vi "JoyStick.vi"(11 "Enum":enum16{"Init", "Run", "End"}(ring)) -> (0 "JoyStick 4":T2, 1 "JoyStick 3":T2, 2 "JoyStick 2":T2, 3 "JoyStick 1":T2)   [LabVIEW 2011]
uses:
  <vilib>/Rock Robotics/WPI/Joystick/WPI_JoystickButtonState.ctl
  <vilib>/Rock Robotics/WPI/Joystick/WPI_JoystickDeviceEnum.ctl
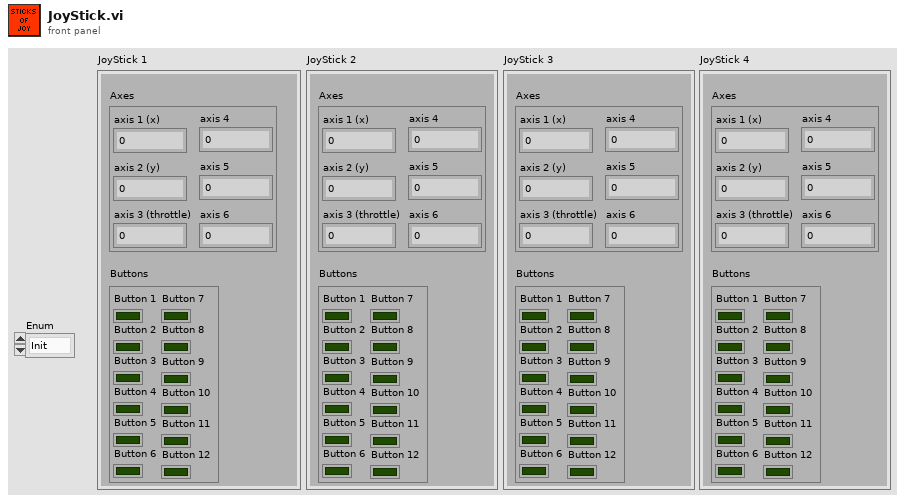
[diagram p1: front panel]
types:
  T1 = typedef "WPI_JoystickButtonState.ctl" = cluster{"Button 1":bool, "Button 2":bool, "Button 3":bool, "Button 4":bool, "Button 5":bool, "Button 6":bool, "Button 7":bool, "Button 8":bool, "Button 9":bool, "Button 10":bool, "Button 11":bool, "Button 12":bool}
  T2 = cluster{"Buttons":T1, "Axes":cluster{"axis 1 (x)":dbl, "axis 2 (y)":dbl, "axis 3 (throttle)":dbl, "axis 4":dbl, "axis 5":dbl, "axis 6":dbl}}
  T3 = typedef "WPI_JoystickDeviceEnum.ctl" = enum16{"USB 1", "USB 2", "USB 3", "USB 4", "Kinect 1", "Kinect 2"}
  T4 = typedef "WPI_JoystickDevRef.ctl" = cluster{"Device":T3}
  T5 = cluster{"axis 1 (x)":dbl, "axis 2 (y)":dbl, "axis 3 (throttle)":dbl, "axis 4":dbl, "axis 5":dbl, "axis 6":dbl}
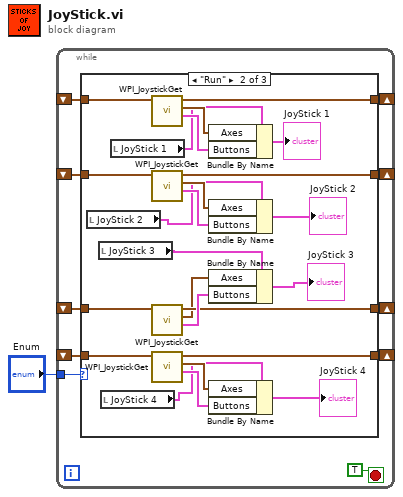
[diagram p0: block diagram]
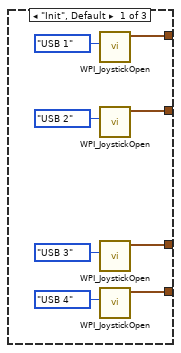
[diagram p2: hidden frame]
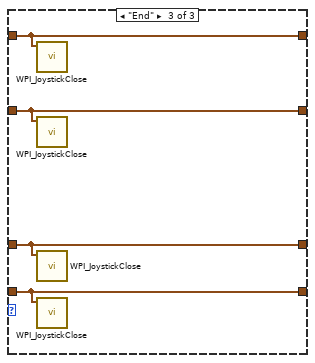
[diagram p3: hidden frame]
diagram:
  n1 = while {
    tunnel: "Enum" -> [w11]
    shift-right: [w10] -> _
    shift-left: _ -> [w8]
    shift-right: [w9] -> _
    shift-left: _ -> [w7]
    shift-right: [w5] -> _
    shift-left: _ -> [w4]
    shift-right: [w6] -> _
    shift-left: _ -> [w3]
    stop <- TRUE stop-if-true
    n2 = case shown="\"Run\"" w11 {
      tunnel: [w19 w42 w47] -> w10
      tunnel: [w18 w30 w46] -> w9
      tunnel: w8 -> [_ w43 w47]
      tunnel: w7 -> [_ w29 w46]
      tunnel: [w17 w26 w44] -> w6
      tunnel: [w16 w33 w45] -> w5
      tunnel: w4 -> [_ w34 w45]
      tunnel: w3 -> [_ w28 w44]
      frame "Init", Default {
        n3 = call <vilib>:"WPI_JoystickOpen.vi"("JoystickDevice"=WPI_JoystickDeviceEnum."USB 1") -> ("JoystickDevRef"=w19:T4)  [unwired: 10 in]
        n4 = call <vilib>:"WPI_JoystickOpen.vi"("JoystickDevice"=WPI_JoystickDeviceEnum."USB 2") -> ("JoystickDevRef"=w18:T4)  [unwired: 10 in]
        n5 = call <vilib>:"WPI_JoystickOpen.vi"("JoystickDevice"=WPI_JoystickDeviceEnum."USB 3") -> ("JoystickDevRef"=w16:T4)  [unwired: 10 in]
        n6 = call <vilib>:"WPI_JoystickOpen.vi"("JoystickDevice"=WPI_JoystickDeviceEnum."USB 4") -> ("JoystickDevRef"=w17:T4)  [unwired: 10 in]
      }
      frame "Run" {
        n7 = local read "JoyStick 2"() -> (w24:T2)
        n8 = local read "JoyStick 3"() -> (w21:T2)
        n9 = local read "JoyStick 4"() -> (w20:T2)
        n10 = local read "JoyStick 1"() -> (w39:T2)
        n11 = call <vilib>:"WPI_JoystickGet.vi"("JoystickDevRef"=w43) -> ("Buttons"=w40:T1, "Axes"=w41:T5, "JoystickDevRef"=w42:T4)  [unwired: 4 in]
        n12 = call <vilib>:"WPI_JoystickGet.vi"("JoystickDevRef"=w29) -> ("Buttons"=w36:T1, "Axes"=w31:T5, "JoystickDevRef"=w30:T4)  [unwired: 4 in]
        n13 = call <vilib>:"WPI_JoystickGet.vi"("JoystickDevRef"=w34) -> ("Buttons"=w35:T1, "Axes"=w32:T5, "JoystickDevRef"=w33:T4)  [unwired: 4 in]
        n14 = call <vilib>:"WPI_JoystickGet.vi"("JoystickDevRef"=w28) -> ("Buttons"=w37:T1, "Axes"=w27:T5, "JoystickDevRef"=w26:T4)  [unwired: 4 in]
        n15 = Bundle By Name(cluster=w39, "Axes"=w41, "Buttons"=w40) -> (→"JoyStick 1":T2)
        n16 = Bundle By Name(cluster=w24, "Axes"=w31, "Buttons"=w36) -> (→"JoyStick 2":T2)
        n17 = Bundle By Name(cluster=w21, "Axes"=w32, "Buttons"=w35) -> (→"JoyStick 3":T2)
        n18 = Bundle By Name(cluster=w20, "Axes"=w27, "Buttons"=w37) -> (→"JoyStick 4":T2)
      }
      frame "End" {
        n19 = call <vilib>:"WPI_JoystickClose.vi"("JoystickDevRef"=w47) -> ()  [unwired: 11 in]
        n20 = call <vilib>:"WPI_JoystickClose.vi"("JoystickDevRef"=w46) -> ()  [unwired: 11 in]
        n21 = call <vilib>:"WPI_JoystickClose.vi"("JoystickDevRef"=w45) -> ()  [unwired: 11 in]
        n22 = call <vilib>:"WPI_JoystickClose.vi"("JoystickDevRef"=w44) -> ()  [unwired: 11 in]
      }
    }
  }
